vi "Save to INI.vi"(8 "error in (no error)":errorcluster, 9 "Create? (T)":bool=TRUE, 10 "INI Path":path, 11 "HAL Manager in":refnum<class "HAL Manager.lvclass">) -> (0 "error out":errorcluster, 3 "HAL Manager out":refnum<class "HAL Manager.lvclass">)   [LabVIEW 2020, in "HAL.lvlib" / "HAL Manager.lvclass"]
uses:
  HAL Manager.lvclass
  HAL Manager.lvclass/HAL Manager.ctl
  Device Config.ctl
  <vilib>/Utility/config.llb/Write Key (String).vi
  <vilib>/Utility/config.llb/Write Key (Path).vi
  Device/Device.lvclass
  <vilib>/Utility/config.llb/NI_LVConfig.lvlib
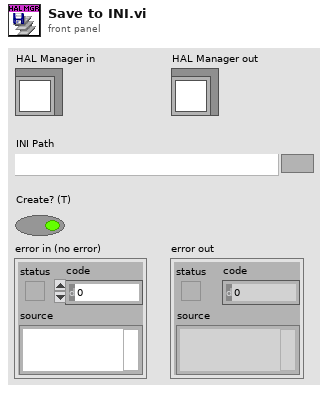
[diagram p1: front panel]
types:
  T1 = typedef "HAL.lvlib/HAL Manager.lvclass/Ref Data.ctl" = cluster{"Devices":refnum<class "Device.lvclass">[], "Type":string[], "Models":string[], "Name":string[]}
  T2 = typedef "HAL.lvlib/HAL Manager.lvclass/Device Config.ctl" = cluster{"Name":string, "Keys":string[], "Values":string[], "Path":path}
  T3 = typedef "NI_LVConfig.lvlib/Config Data RefNum.ctl" = refnum<k1>
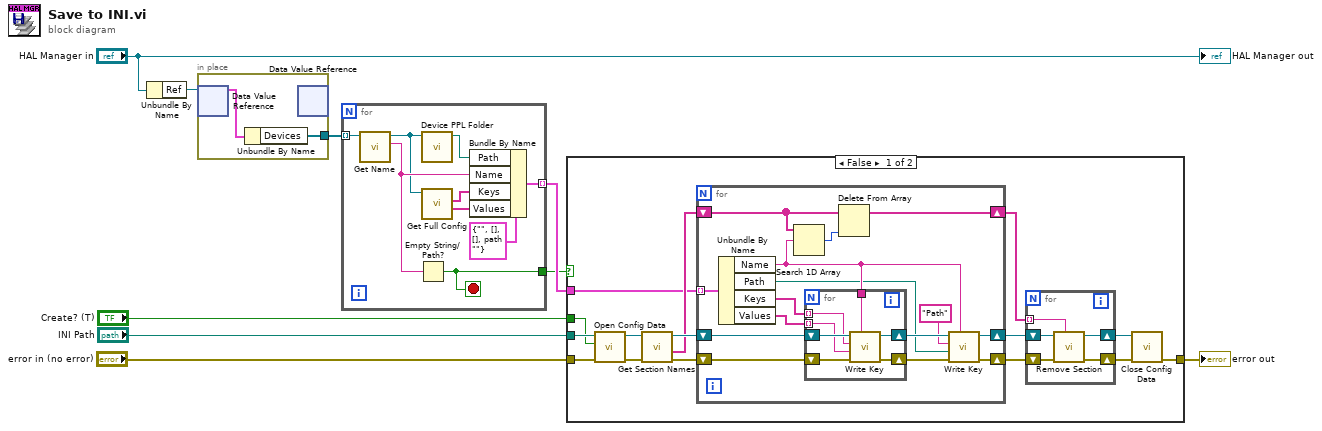
[diagram p0: block diagram]
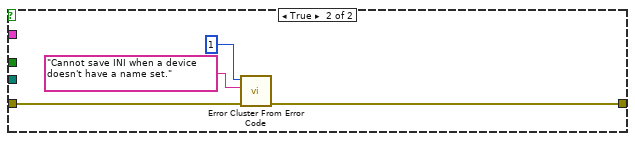
[diagram p2: hidden frame]
diagram:
  n1 = Unbundle By Name("HAL Manager in") -> ("Ref"=w9:refnum<data-value>)
  n2 = in-place {
    in-place-border: [w10] -> w7
    n3 = in-place-dvr #1(w9) -> (w11:T1)  [unwired: 1 out]
    n4 = Unbundle By Name(w11) -> ("Devices"=w10:refnum<class "Device.lvclass">[])
    n5 = in-place-dvr #1() -> ()  [unwired: 1 in, 2 out]
  }
  n6 = for {
    tunnel: w7 -> [w20] mode=indexing
    tunnel: [w15] -> w1
    tunnel: [w14] -> w6 mode=indexing
    stop <- w15 stop-if-true
    n7 = call "Get Name.vi"("Device in"=w20) -> ("Name"=w16:string, "Device out"=w13:refnum<class "Device.lvclass">)  [unwired: 8 in, 1 out]
    n8 = Empty String/Path?(string/path=w16) -> (empty?=w15:bool)
    n9 = call "Device PPL Folder.vi"("Device in"=w13) -> ("Relative Class Path"=w12:path)  [unwired: 7 in, 3 out]
    n10 = call "Get Full Config.vi"("Device in"=w13) -> ("Config Values"=w17:string[], "Config Keys"=w18:string[])  [unwired: 7 in, 2 out]
    n11 = Bundle By Name(cluster=T2 {"Name"="", "Keys"=[], "Values"=[], "Path"=path ""} ("Device Config"), "Path"=w12, "Name"=w16, "Keys"=w18, "Values"=w17) -> (w14:T2)
  }
  n12 = case shown="False" w1 {
    tunnel: w6 -> [w27 _]
    tunnel: "error in (no error)" -> [w35 w65]
    tunnel: "INI Path" -> [w34 _]
    tunnel: "Create? (T)" -> [w33 _]
    tunnel: [w21 w64] -> w2
    frame False {
      n13 = call <vilib>:"Open Config Data.vi"("error in (no error)"=w35, "create file if necessary (T)"=w33, "configuration file path"=w34) -> ("error out"=w31:errorcluster, "refnum"=w32:T3)  [unwired: 6 in, 1 out]
      n14 = call <vilib>:"Get Section Names.vi"("error in (no error)"=w31, "refnum"=w32) -> ("error out"=w30:errorcluster, "section names"=w28:string[], "refnum out"=w29:T3)  [unwired: 7 in]
      n15 = for {
        shift-right: [w37] -> w25
        shift-left: w29 -> [w49]
        shift-right: [w36] -> w26
        shift-left: w30 -> [w48]
        shift-right: [w43] -> w24
        shift-left: w28 -> [w45]
        tunnel: w27 -> [w50] mode=indexing
        n16 = Unbundle By Name(w50) -> ("Name"=w40:string, "Path"=w39:path, "Keys"=w47:string[], "Values"=w46:string[])
        n17 = Search 1D Array(1D array=w45, element=w40) -> (index of element=w44:i32)  [unwired: 1 in]
        n18 = for {
          tunnel: w40 -> [w56]
          shift-right: [w52] -> w42
          shift-left: w49 -> [w57]
          shift-right: [w51] -> w41
          shift-left: w48 -> [w55]
          tunnel: w47 -> [w54] mode=indexing
          tunnel: w46 -> [w53] mode=indexing
          n19 = call-poly <vilib>:"Write Key.vi"("section"=w56, "error in (no error)"=w55, "value"=w53, "key"=w54, "refnum"=w57) -> ("error out"=w51:errorcluster, "refnum out"=w52:T3)  [unwired: 4 in, 1 out]
        }
        n20 = Delete From Array(array=w45, index=w44) -> (array with subset deleted=w43:string[])  [unwired: 1 in, 1 out]
        n21 = call-poly <vilib>:"Write Key.vi"("section"=w40, "error in (no error)"=w41, "value"=w39, "key"="Path", "refnum"=w42) -> ("error out"=w36:errorcluster, "refnum out"=w37:T3)  [unwired: 4 in, 1 out]
      }
      n22 = for {
        shift-right: [w58] -> w22
        shift-left: w26 -> [w61]
        shift-right: [w59] -> w23
        shift-left: w25 -> [w62]
        tunnel: w24 -> [w60] mode=indexing
        n23 = call <vilib>:"Remove Section.vi"("section"=w60, "error in (no error)"=w61, "refnum"=w62) -> ("error out"=w58:errorcluster, "refnum out"=w59:T3)  [unwired: 6 in, 1 out]
      }
      n24 = call <vilib>:"Close Config Data.vi"("error in (no error)"=w22, "refnum"=w23) -> ("error out"=w21:errorcluster)  [unwired: 8 in, 1 out]
    }
    frame True {
      n25 = call <vilib>:"Error Cluster From Error Code.vi"("error in (no error)"=w65, "error message (\"\")"="Cannot save INI when a device doesn't have a name set." ("error message (\"\")"), "error code (0)"=1) -> ("error out"=w64:errorcluster)  [unwired: 6 in]
    }
  }
  "error out" <- w2
  "HAL Manager out" <- "HAL Manager in"
